vi "LowPass Filter.vi"(1 "Filter Input":dbl, 2 "Ts [s]":dbl) -> (0 "Filter Output":dbl)   [LabVIEW 2022 SP3]
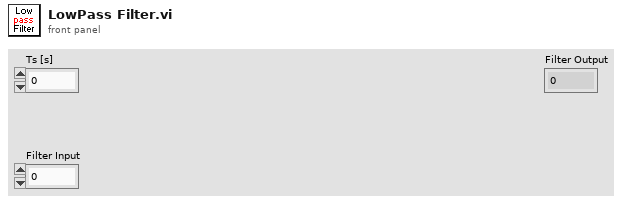
[diagram p1: front panel]
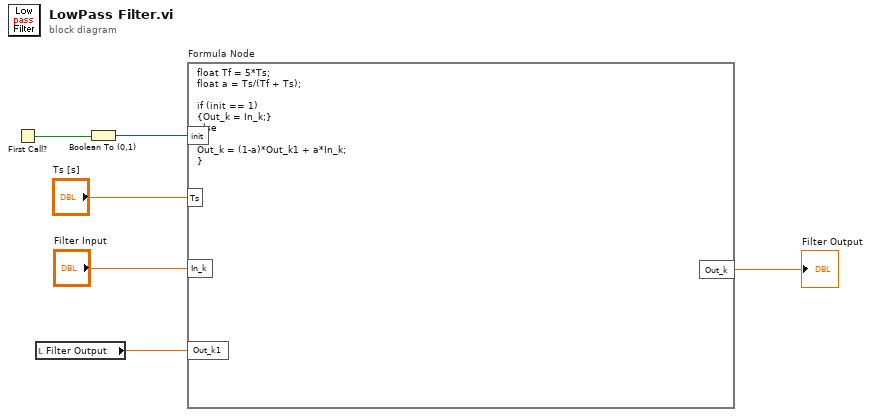
[diagram p0: block diagram]
diagram:
  n1 = First Call?() -> (First Call?: T/F=w6:bool)
  n2 = local read "Filter Output"() -> (w1:dbl)
  n3 = Boolean To (0,1)(Boolean=w6) -> (0, 1=w5:i16)
  n4 = formula code="float Tf = 5*Ts;\nfloat a = Ts/(Tf + Ts);\n\nif (init == 1)\n{Out_k = In_k;}\nelse\n{\nOut_k = (1-a)*Out_k1 + a*In_k;\n}"("init"=w5, "Ts"="Ts [s]", "In_k"="Filter Input", "Out_k1"=w1) -> ("Out_k"=→"Filter Output":dbl)
